vi "Configure.vi"(8 "error in (no error)":errorcluster, 11 "RF Powers in":refnum<class "RF Power.lvclass">) -> (0 "error out":errorcluster, 3 "RF Powers out":refnum<class "RF Power.lvclass">)   [LabVIEW 2020, in "RF Power.lvclass"]
doc: "Configure the measurements paramaters to sweep.\nThis should be a pop up interface invoked by the configure test button on the main panel."
uses:
  RF Power.lvclass
  Controls/Loop order.ctl
  Controls/Config info.ctl
panel:
  in  "SG":i32=1 caption="Signal Generator #" min=1 max=2 step=1
  in  "Power Meter \npath loss compensation":bool=TRUE
  in  "Signal Generator \npath loss compensation":bool=TRUE
  in  "Loop order":T1
  in  "Cancel Button":bool
  in  "OK Button":bool
  in  "Power (dBm)":string="-20"
  in  "Frequency (MHz)":string="900"
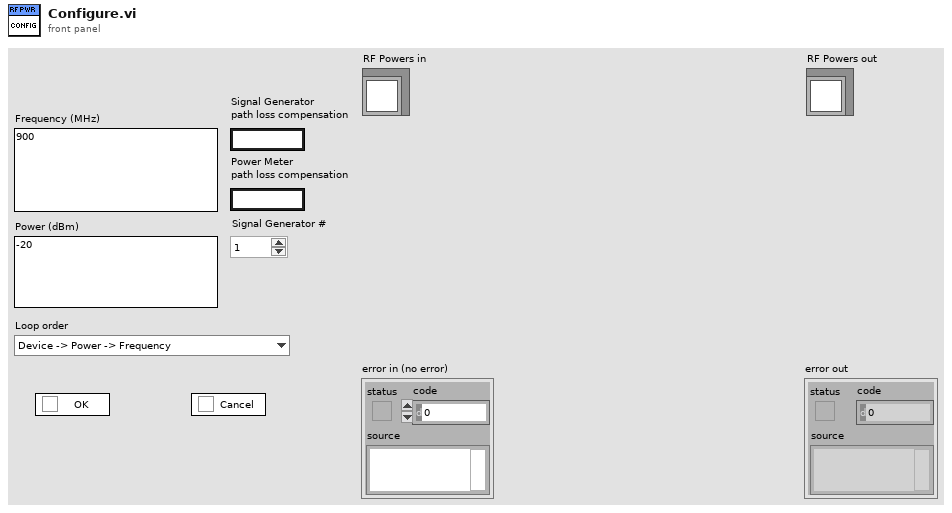
[diagram p1: front panel]
types:
  T1 = typedef "RF Power.lvclass/Loop order.ctl" = enum16{"Device -> Power -> Frequency", "Device -> Frequency -> Power"}
  T2 = typedef "RF Power.lvclass/Config info.ctl" = cluster{"Frequency (MHz)":string, "Power (dBm)":string, "Loop order":T1, "SG loss":bool, "PM loss":bool, "SG":i32}
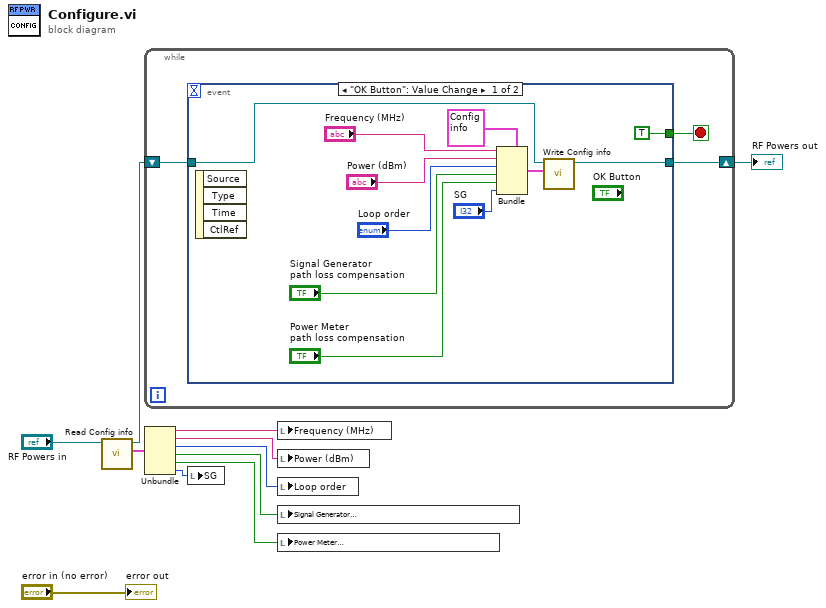
[diagram p0: block diagram]
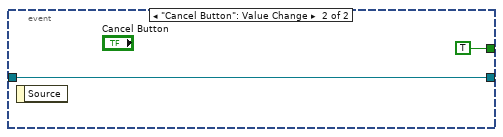
[diagram p2: hidden frame]
diagram:
  n1 = call-dynamic "Read Config info.vi"("RF Power in"="RF Powers in") -> ("Config info"=w7:T2, "RF Power out"=w8:refnum<class "RF Power.lvclass">)  [unwired: 9 in]
  n2 = while {
    shift-right: [w13] -> w11
    shift-left: w8 -> [w14]
    stop <- w12 stop-if-true
    n3 = event shown="[0] \"OK Button\": Value Change" {
      selector: _ -> [_ _]
      dyn-events: _ -> [_ _]
      timeout: _ -> [_ _]
      tunnel: w14 -> [w21 w26]
      tunnel: [w20 w26] -> w13
      tunnel: [TRUE TRUE] -> w12
      event "OK Button": Value Change {
        n4 = event-data() -> ()  [unwired: 1 in, 4 out]
        n5 = Bundle(cluster=T2 {"Frequency (MHz)"="", "Power (dBm)"="", "Loop order"=enum."Device -> Power -> Frequency", "SG loss"=TRUE, "PM loss"=TRUE, "SG"=1} ("Config info"), "Frequency (MHz)"="Frequency (MHz)", "Power (dBm)"="Power (dBm)", "Loop order"="Loop order", "SG loss"="Signal Generator \npath loss compensation", "PM loss"="Power Meter \npath loss compensation", "SG"="SG") -> (w22:T2)
        n6 = call-dynamic "Write Config info.vi"("Config info"=w22, "RF Power in"=w21) -> ("RF Power out"=w20:refnum<class "RF Power.lvclass">)  [unwired: 9 in]
      }
      event "Cancel Button": Value Change {
        n7 = event-data() -> ()  [unwired: 1 in, 1 out]
      }
    }
  }
  "RF Powers out" <- w11
  n8 = Unbundle(w7) -> ("Frequency (MHz)"=w1:string, "Power (dBm)"=w2:string, "Loop order"=w3:T1, "SG loss"=w4:bool, "PM loss"=w5:bool, "SG"=w6:i32)
  n9 = local write "SG"(w6) -> ()
  n10 = local write "Frequency (MHz)"(w1) -> ()
  n11 = local write "Power (dBm)"(w2) -> ()
  n12 = local write "Loop order"(w3) -> ()
  n13 = local write "Signal Generator \npath loss compensation"(w4) -> ()
  n14 = local write "Power Meter \npath loss compensation"(w5) -> ()
  "error out" <- "error in (no error)"
